vi "ServoTest.vi"() -> ()   [LabVIEW 2017]
panel:
  in  "Select Channel":string(combo)="Servo 1"
  in  "Set Servo Position (0 - 180 degrees)":u8(slide)=90 scale=0.0..180.0
  out "Servo Position":u8
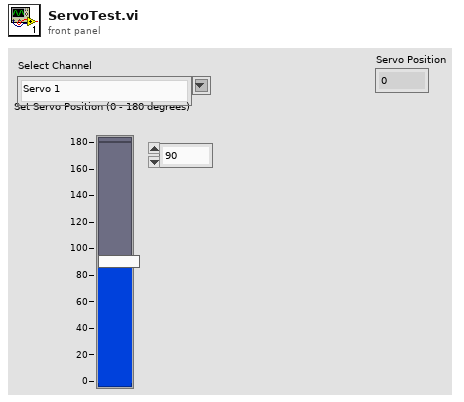
[diagram p1: front panel]
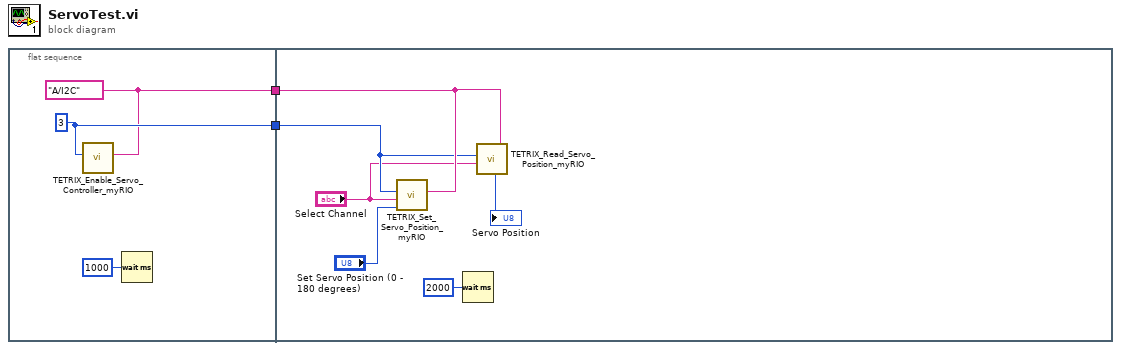
[diagram p0: block diagram]
diagram:
  n1 = flat-sequence {
    tunnel: [w3] -> w2
    tunnel: [w4] -> w1
    tunnel: w2 -> [w9]
    tunnel: w1 -> [w8]
    frame #0 {
      w4 = u8 3 ("Controller ID#  (I2C Address)")
      w3 = tag "A/I2C" ("myRIO MXP Port A/B")
      n2 = call <vilib>:"TETRIX_Enable_Servo_Controller_myRIO.vi"("myRIO MXP Port A/B"=w3, "Controller ID#  (I2C Address)"=w4) -> ()  [unwired: 5 in, 1 out]
      n3 = Wait (ms)(milliseconds to wait=u32 1000) -> ()  [unwired: 1 out]
    }
    frame #1 {
      n4 = call <vilib>:"TETRIX_Set_Servo_Position_myRIO.vi"("myRIO MXP Port A/B"=w9, "Set Servo Position (0 - 180 degrees)"="Set Servo Position (0 - 180 degrees)", "Select Channel"="Select Channel", "Controller ID#  (I2C Address)"=w8) -> ()  [unwired: 3 in, 1 out]
      n5 = Wait (ms)(milliseconds to wait=u32 2000) -> ()  [unwired: 1 out]
      n6 = call <vilib>:"TETRIX_Read_Servo_Position_myRIO.vi"("myRIO MXP Port A/B"=w9, "Select Channel"="Select Channel", "Controller ID#  (I2C Address)"=w8) -> ("Servo Position"=→"Servo Position":u8)  [unwired: 3 in, 1 out]
    }
  }
